vi "Sin Gen Test.vi"() -> ()   [LabVIEW 2012]
uses:
  <vilib>/rvi/FXPMathLib/basic elements/FxpIntAccumulator/subVIs/nifxpmath_IntAccumulator_SimConfig.ctl
  <vilib>/rvi/FXPMathLib/FxpSinAndCos/subVIs/nifxpmath_SinAndCos_SimConfig.ctl
  <vilib>/rvi/FXPMathLib/basic elements/FxpIntAccumulator/simVIs/DllFxpIntAccumulator_sub.vi
  <vilib>/rvi/FXPMathLib/FxpSinAndCos/simVIs/DllFxpSinAndCosTemp_sub.vi
  <vilib>/rvi/eio/common/nirviEmuTemplateMethod_errors.vi
  <vilib>/rvi/FXPMathLib/basic elements/FxpIntAccumulator/XNode/nifxpmath_IntAccumulator.xnode
  <vilib>/rvi/FXPMathLib/FxpSinAndCos/XNode/nifxpmath_SinAndCos.xnode
  <vilib>/rvi/FXPMathLib/FxpMul/XNode/nifxpmath_Multiplier.xnode
  <vilib>/eio/EIONode/EIONode.xnode
  <vilib>/rvi/FXPMathLib/sim/FxpSim.dll
panel:
  out "Numeric 2":fxp<+/-,64,32>
  in  "Voltage (V)":fxp<+/-,32,16>
  in  "Numeric":fxp<+/-,64,32>
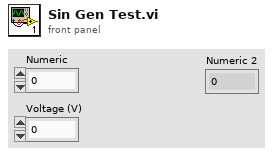
[diagram p1: front panel]
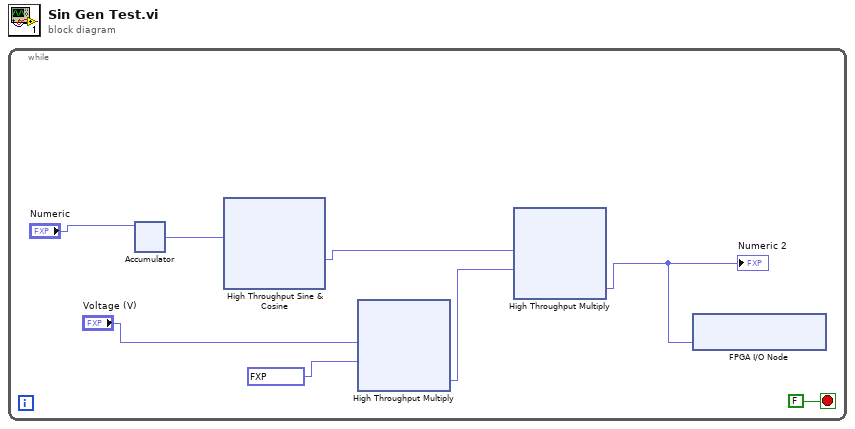
[diagram p0: block diagram]
diagram:
  n1 = while {
    stop <- FALSE stop-if-true
    n2 = xnode "Accumulator"("x"="Numeric") -> ("s"=w6:fxp<+/-,64,32>)  [unwired: 4 in, 1 out]
    n3 = xnode "High Throughput Sine & Cosine"("x (pi)"=w6) -> ("sin(x)"=w4:fxp<+/-,16,2>)  [unwired: 1 out]
    n4 = xnode ("High Throughput Multiply")("x"="Voltage (V)", "y"=fxp<+,16,12> 3276.8125) -> ("x*y"=w5:fxp<+/-,48,28>)
    n5 = xnode ("High Throughput Multiply")("x"=w4, "y"=w5) -> ("x*y"=w1:fxp<+/-,64,30>)
    "Numeric 2" <- w1
    n6 = xnode "FPGA I/O Node"("Connector0/AO4"=w1) -> ()  [unwired: 1 in, 1 out]
  }
